vi "update stimulator odor colors (sub-vi).vi"(8 "error in (no error)":errorcluster, 9 "changed? [] (empty, all true)":bool[](array[boolean]), 10 "odor-color map":T1, 11 "stim. config array refnum":refnum<vi>) -> (0 "error out":errorcluster, 3 "stim. config array refnum out":refnum<vi>, 4 "value error":errorcluster)   [LabVIEW 2021]
uses:
  type-defs/stimulation configuration array (type def).ctl
  type-defs/stimulator configuration line cluster (type def).ctl
  type-defs/port-odor with color cluster (type def).ctl
  type-defs/port-odor ring (type def).ctl
  type-defs/odor color (type def).ctl
  type-defs/odor channel to odor color map (type def).ctl
  type-defs/odor selection (type def).ctl
  type-defs/odor color enum (type def).ctl
  <vilib>/Utility/error.llb/Error Cluster From Error Code.vi
  <vilib>/ErrorRing/Error Ring.xnode
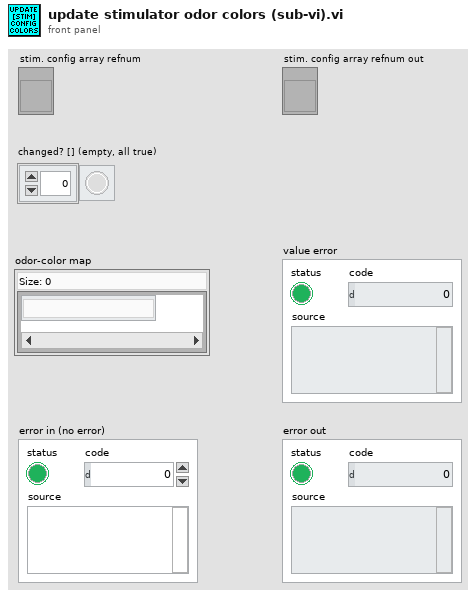
[diagram p1: front panel]
types:
  T1 = typedef "odor channel to odor color map (type def).ctl" = map{T2, T3}
  T2 = typedef "odor selection (type def).ctl" = enum16{"[none]", "odor 1", "odor 2", "odor 3", "odor 4", "odor 5", "odor 6", "odor 7", "odor 8", "odor 9", "odor 10"}
  T3 = typedef "odor color (type def).ctl" = u16
  T4 = typedef "odor color enum (type def).ctl" = enum16{"white", "blue", "red", "orange", "yellow", "green", "magenta", "brown", "black", "[none]"}
  T5 = typedef "stimulation configuration array (type def).ctl" = T6[]
  T6 = typedef "stimulator configuration line cluster (type def).ctl" = cluster{"description":string, "duration, s":dbl, "left odor":T7, "middle odor":T7, "right odor":T7, "selected?":bool}
  T7 = typedef "port-odor with color cluster (type def).ctl" = cluster{"port-odor ring":T8, "odor color":T3}
  T8 = typedef "port-odor ring (type def).ctl" = u16
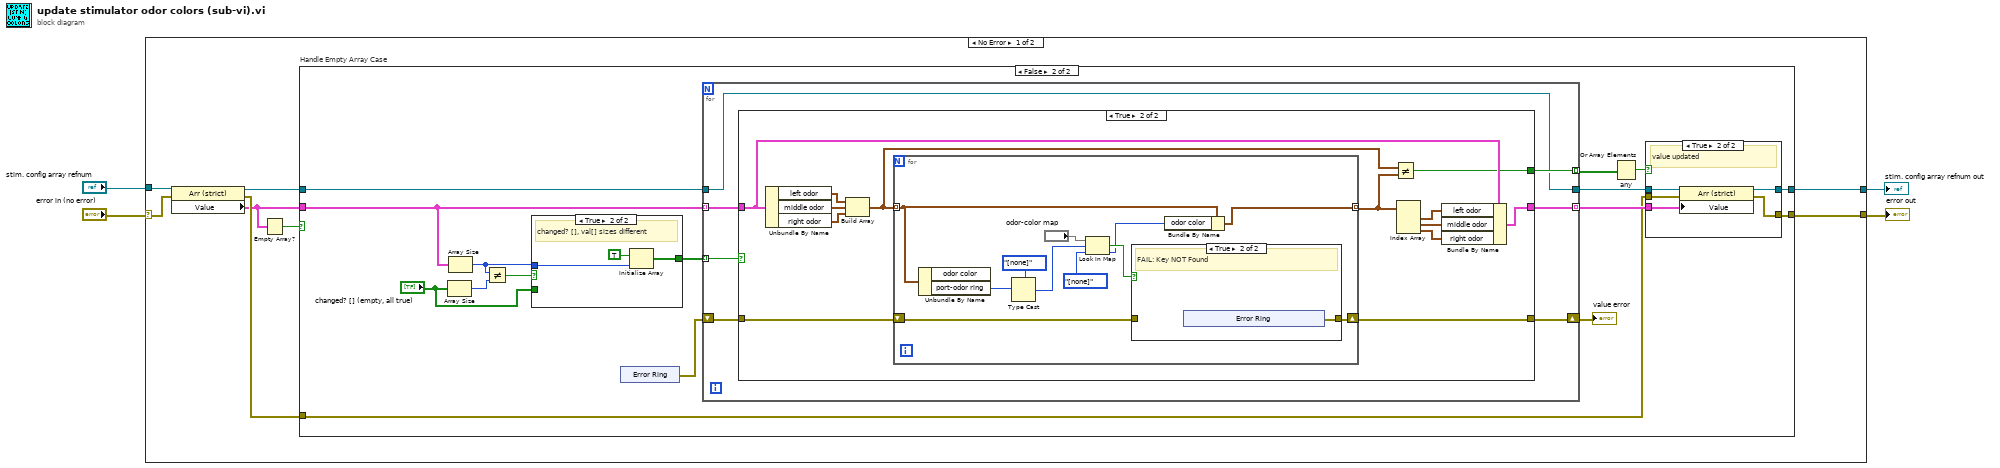
[diagram p0: block diagram]
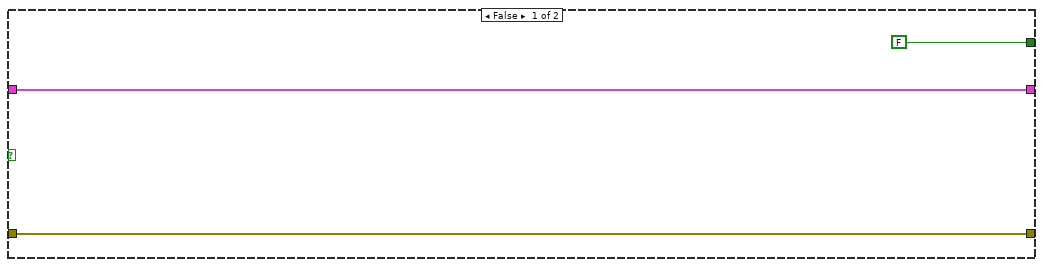
[diagram p5: hidden frame]
diagram:
  n1 = case shown="No Error" "error in (no error)" {
    selector: "error in (no error)" -> [w10 w85]
    tunnel: "stim. config array refnum" -> [w12 w84]
    tunnel: [w9 w84] -> w2
    tunnel: [w8 w85] -> w1
    frame No Error {
      n2 = property class="Arr (strict)"(reference=w12, error in=w10) -> (reference out=w11:refnum<vi>, error out=w7:errorcluster, "Value"=w6:T5)
      n3 = Empty Array?(array=w6) -> (empty?=w5:bool)
      n4 = case "Handle Empty Array Case" shown="False" w5 {
        tunnel: w11 -> [w14 w30]
        tunnel: [w14 w27] -> w9
        tunnel: [w13 w26] -> w8
        tunnel: w6 -> [_ w19]
        tunnel: w7 -> [w13 w25]
        frame True {
        }
        frame False {
          n5 = Array Size(array="changed? [] (empty, all true)") -> (size(s)=w18:i32)
          n6 = Array Size(array=w19) -> (size(s)=w17:i32)
          n7 = Not Equal?(x=w17, y=w18) -> (x != y?=w20:bool)
          n8 = case shown="True" w20 {
            tunnel: w17 -> [_ w34]
            tunnel: [w31 w32] -> w16
            tunnel: "changed? [] (empty, all true)" -> [w31 _]
            frame False {
              # "changed? [], val[] sizes same"
            }
            frame True {
              # "changed? [], val[] sizes different"
              n9 = Initialize Array(TRUE, w34) -> (w32:bool[])
            }
          }
          n10 = xnode "Error Ring"() -> ("error out"=w23:errorcluster)
          n11 = for {
            tunnel: w19 -> [w47] mode=indexing
            tunnel: w30 -> [w43]
            shift-right: [w48] -> w24
            shift-left: w23 -> [w49]
            tunnel: [w46] -> w29 mode=indexing
            tunnel: [w43] -> w28
            tunnel: w16 -> [w44] mode=indexing
            tunnel: [w45] -> w22 mode=indexing
            n12 = case shown="True" w44 {
              tunnel: w49 -> [w50 w62]
              tunnel: [w50 w61] -> w48
              tunnel: w47 -> [w51 w60]
              tunnel: [w51 w58] -> w46
              tunnel: [FALSE w53] -> w45
              frame False {
              }
              frame True {
                n13 = Unbundle By Name(w60) -> ("left odor"=w65:T7, "middle odor"=w64:T7, "right odor"=w63:T7)
                n14 = Build Array(w65, w64, w63) -> (w55:T7[])
                n15 = for {
                  tunnel: w55 -> [w71] mode=indexing
                  shift-right: [w67] -> w61
                  shift-left: w62 -> [w66]
                  tunnel: [w68] -> w54 mode=indexing
                  n16 = Unbundle By Name(w71) -> ("port-odor ring"=w76:T8)  [unwired: 1 out]
                  n17 = Type Cast(type=odor_selection_(type_def)."[none]" ("Enum"), x=w76) -> (*(type *) &x=w73:T2)
                  n18 = Look In Map(map="odor-color map", key=w73, default value=odor_color_enum_(type_def)."[none]" ("Enum")) -> (key not found?=w72:bool, value=w69:T3)
                  n19 = case shown="True" w72 {
                    tunnel: [w77 w78] -> w67
                    tunnel: w66 -> [w77 _]
                    frame False {
                      # "SUCCESS: Key Found"
                    }
                    frame True {
                      # "FAIL: Key NOT Found"
                      n20 = xnode "Error Ring"() -> ("error out"=w78:errorcluster)
                    }
                  }
                  n21 = Bundle By Name(cluster=w71, "odor color"=w69) -> (w68:T7)
                }
                n22 = Not Equal?(x=w55, y=w54) -> (x != y?=w53:bool)
                n23 = Index Array(array=w54) -> (element #1=w59:T7, element #2=w57:T7, element #3=w56:T7)  [unwired: 3 in]
                n24 = Bundle By Name(cluster=w60, "left odor"=w59, "middle odor"=w57, "right odor"=w56) -> (w58:T6)
              }
            }
          }
          "value error" <- w24
          n25 = Or Array Elements "any"(Boolean array=w22) -> (logical OR=w21:bool)
          n26 = case shown="True" w21 {
            tunnel: w29 -> [_ w41]
            tunnel: w28 -> [w35 w40]
            tunnel: [w35 w39] -> w27
            tunnel: [w36 w38] -> w26
            tunnel: w25 -> [w36 w37]
            frame False {
              # "value unchanged"
            }
            frame True {
              # "value updated"
              n27 = property class="Arr (strict)"(reference=w40, error in=w37, "Value"=w41) -> (reference out=w39:refnum<vi>, error out=w38:errorcluster)
            }
          }
        }
      }
    }
    frame Error {
    }
  }
  "stim. config array refnum out" <- w2
  "error out" <- w1
